vi "get_thermocouple_calibration_type.vi"(8 "error in (no error)":errorcluster, 11 "connection ID":refnum<k5>) -> (0 "error out":errorcluster, 2 "Thermocouple calibration type":T1, 3 "connection ID out":refnum<k5>)   [LabVIEW 2018]
uses:
  typedefs/thermocouple_calibration_types.ctl
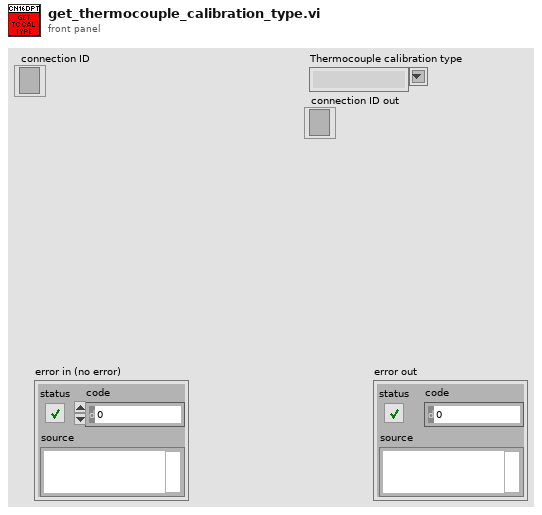
[diagram p1: front panel]
types:
  T1 = typedef "thermocouple_calibration_types.ctl" = string
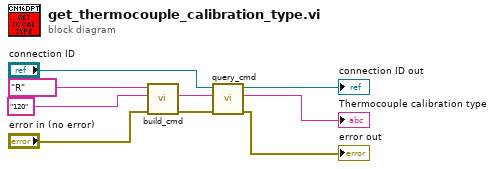
[diagram p0: block diagram]
diagram:
  n1 = call "build_cmd.vi"("error in (no error)"="error in (no error)", "Command ID"="120", "Command class"="R") -> ("error out"=w5:errorcluster, "Command"=w4:string)  [unwired: 7 in]
  n2 = call "query_cmd.vi"("error in (no error)"=w5, "Command"=w4, "connection ID"="connection ID") -> ("error out"=→"error out":errorcluster, "Response"=→"Thermocouple calibration type":string, "connection ID out"=→"connection ID out":refnum<k5>)  [unwired: 6 in]
